vi "WT300 Collect Raw Data.vi"(6 "Timeout (10000 ms)":i32=1000, 8 "error in (no error)":errorcluster, 11 "VISA Refnum in":refnum<visa-resource-name>) -> (0 "error out":errorcluster, 1 "Headers":string[](array[string]), 2 "Data":dbl[](array[numeric]), 3 "VISA resource name out":refnum<visa-resource-name>)   [LabVIEW 2023]
uses:
  <vilib>/Utility/error.llb/whitespace.ctl
  <vilib>/Utility/error.llb/Trim Whitespace One-Sided.vi
  Public/Data/Read Measurement (Normal).vi
  Yokogawa WT300 Series.lvlib
panel:
  out "Array":bool[](array[boolean])
  out "All Headers Match":bool
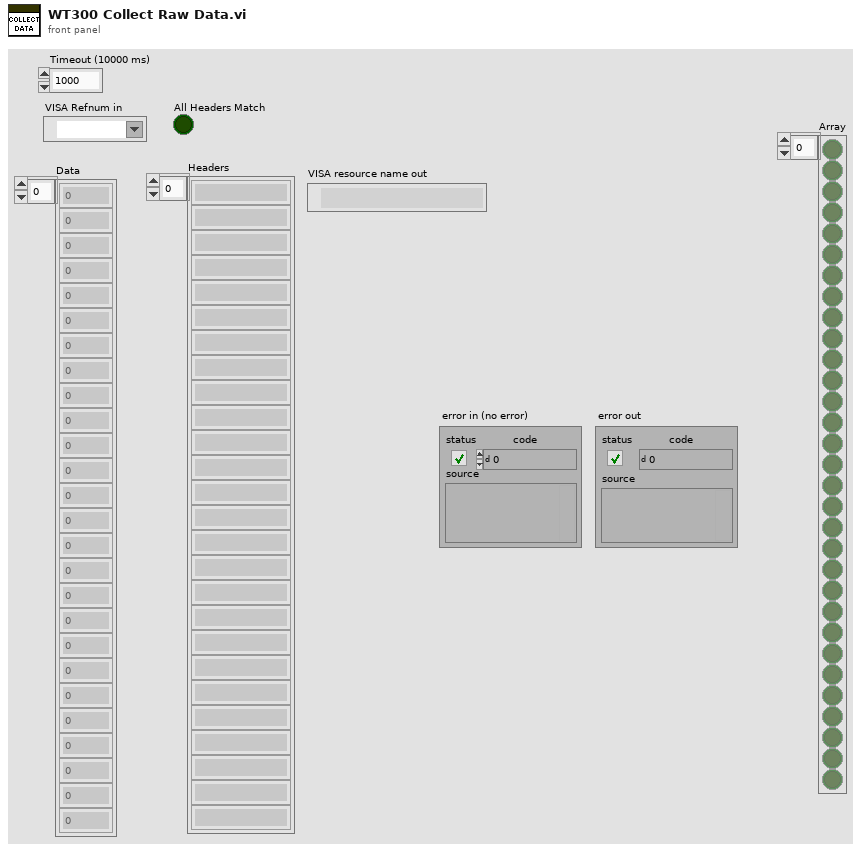
[diagram p1: front panel]
types:
  T1 = typedef "whitespace.ctl" = u16
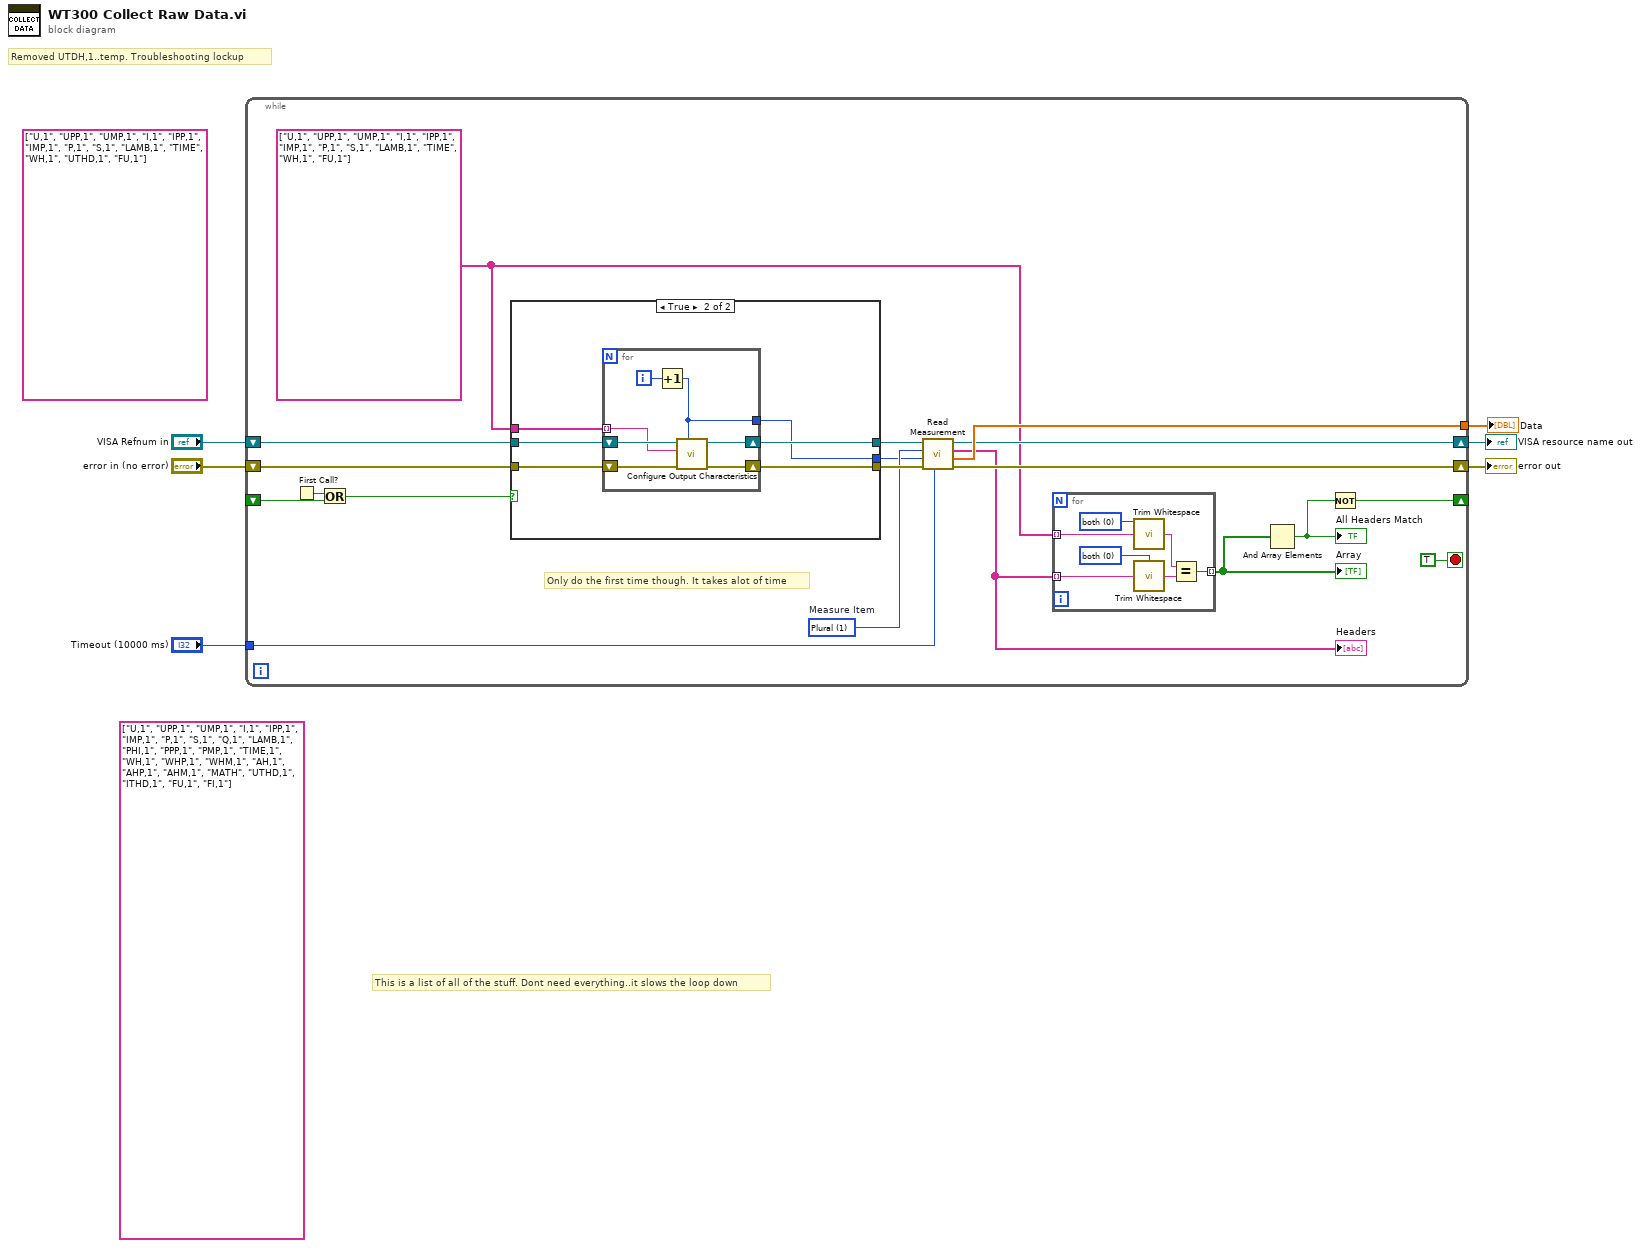
[diagram p0: block diagram]
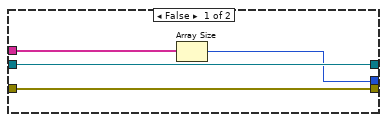
[diagram p2: hidden frame]
diagram:
  (unwired) string[] ["U,1", "UPP,1", "UMP,1", "I,1", "IPP,1", "IMP,1", "P,1", "S,1", "LAMB,1", "TIME", "WH,1", "UTHD,1", "FU,1"] ("appended array 2")
  (unwired) string[] ["U,1", "UPP,1", "UMP,1", "I,1", "IPP,1", "IMP,1", "P,1", "S,1", "Q,1", "LAMB,1", "PHI,1", "PPP,1", "PMP,1", "TIME,1", "WH,1", "WHP,1", "WHM,1", "AH,1", "AHP,1", "AHM,1", "MATH", "UTHD,1", "ITHD,1", "FU,1", "FI,1"] ("appended array 2")
  # "Removed UTDH,1..temp. Troubleshooting lockup"
  # "This is a list of all of the stuff. Dont need everything..it slows the loop down"
  n1 = while {
    tunnel: [w21] -> w5
    shift-right: [w19] -> w4
    shift-left: "VISA Refnum in" -> [w25]
    shift-right: [w18] -> w3
    shift-left: "error in (no error)" -> [w17]
    shift-right: [w11] -> _
    shift-left: _ -> [w9]
    tunnel: "Timeout (10000 ms)" -> [w7]
    stop <- TRUE stop-if-true
    w14 = string[] ["U,1", "UPP,1", "UMP,1", "I,1", "IPP,1", "IMP,1", "P,1", "S,1", "LAMB,1", "TIME", "WH,1", "FU,1"] ("appended array 2")
    w22 = 1 items=["One", "Plural"]  # Measure Item
    # "Only do the first time though. It takes alot of time"
    n2 = First Call?() -> (First Call?: T/F=w10:bool)
    n3 = Or(x=w10, y=w9) -> (x .or. y?=w8:bool)
    n4 = case shown="True" w8 {
      tunnel: w14 -> [w34 w42]
      tunnel: w25 -> [w36 w41]
      tunnel: [w36 w40] -> w24
      tunnel: [w35 w39] -> w23
      tunnel: [w33 w38] -> w20
      tunnel: w17 -> [w35 w37]
      frame False {
        n5 = Array Size(array=w34) -> (size(s)=w33:i32)
      }
      frame True {
        n6 = for {
          shift-right: [w49] -> w40
          shift-left: w41 -> [w45]
          shift-right: [w48] -> w39
          shift-left: w37 -> [w46]
          tunnel: w42 -> [w44] mode=indexing
          tunnel: [w43] -> w38
          i -> [w47]
          n7 = Increment(x=w47) -> (x+1=w43:i32)
          n8 = call "Configure Output Characteristics.vi"("Item (1)"=w43, "error in (no error)"=w46, "Function (Empty)"=w44, "VISA resource name"=w45) -> ("error out"=w48:errorcluster, "VISA resource name out"=w49:refnum<visa-resource-name>)  [unwired: 6 in]
        }
      }
    }
    n9 = call-poly "Read Measurement.vi"("Timeout (10000 ms)"=w7, "error in (no error)"=w23, "Number of Item (15)"=w20, "Measure Item (1: Plural)"=w22, "VISA resource name"=w24) -> ("error out"=w18:errorcluster, "Measurement"=w21:dbl[], "Function"=w15:string[], "VISA resource name out"=w19:refnum<visa-resource-name>)  [unwired: 3 in]
    "Headers" <- w15
    n10 = for {
      tunnel: w15 -> [w28] mode=indexing
      tunnel: w14 -> [w31] mode=indexing
      tunnel: [w32] -> w13 mode=indexing
      w26 = T1 0 items=["both", "start of string", "end of string"] ("location (both)")
      w27 = T1 0 items=["both", "start of string", "end of string"] ("location (both)")
      n11 = call <vilib>:"Trim Whitespace.vi"("string"=w31, "location (both)"=w27) -> ("trimmed string"=w30:string)
      n12 = call <vilib>:"Trim Whitespace.vi"("string"=w28, "location (both)"=w26) -> ("trimmed string"=w29:string)
      n13 = Equal?(x=w30, y=w29) -> (x = y?=w32:bool)
    }
    "Array" <- w13
    n14 = And Array Elements(Boolean array=w13) -> (logical AND=w12:bool)
    "All Headers Match" <- w12
    n15 = Not(x=w12) -> (.not. x?=w11:bool)
  }
  "Data" <- w5
  "VISA resource name out" <- w4
  "error out" <- w3
